vi "lvEtherbone.sdb_find_by_address.vi"(0 "eb_socket_ID":i32, 1 "eb_device_ID":i32, 2 "address":u64 format="%.0x", 5 "error in (no error)":errorcluster) -> (10 "addr_first":u64 format="%.0x", 12 "addr_last":u64 format="%.0x", 13 "eb_status":T1 items=["EB_SUCCESS"=1, "EB_OK"=0, "EB_FAIL"=-1, "EB_ADDRESS"=-2, "EB_WIDTH"=-3, "EB_OVERFLOW"=-4, "EB_ENDIAN"=-5, "EB_BUSY"=-6, "EB_TIMEOUT"=-7, "EB_OOM"=-8, "EB_ABI"=-9, "EB_SEGFAULT"=-10], 14 "eb_socket_ID out":i32, 15 "eb_device_ID out":i32, 16 "vendor_id":u64 format="%.0x", 17 "device_id":u32 format="%.0x", 18 "name":string, 19 "error out":errorcluster)   [LabVIEW 2012, in "lvEtherbone.lvlib"]
doc: "/* Find the SDB record for a device at address.\n * If no matching record is found EB_ADDRESS is returned.\n * On success, EB_OK is returned.\n * Other failures are possible.\n */\nEB_PUBLIC eb_status_t eb_sdb_find_by_address(eb_device_t device, eb_address_t address, struct sdb_device* output);"
uses:
  lvEtherbone.lvlib
  lvEtherbone.lveb_status_t.ctl
  libetherbone.so
panel:
  in  "eb_status_t":T1 items=["EB_SUCCESS"=1, "EB_OK"=0, "EB_FAIL"=-1, "EB_ADDRESS"=-2, "EB_WIDTH"=-3, "EB_OVERFLOW"=-4, "EB_ENDIAN"=-5, "EB_BUSY"=-6, "EB_TIMEOUT"=-7, "EB_OOM"=-8, "EB_ABI"=-9, "EB_SEGFAULT"=-10]
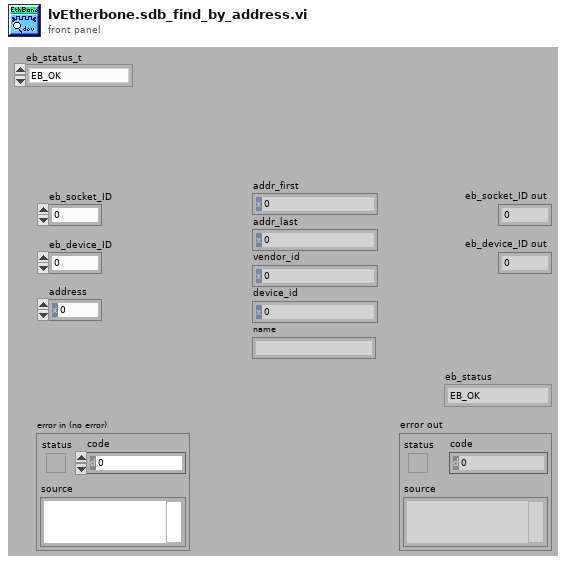
[diagram p1: front panel]
types:
  T1 = typedef "lvEtherbone.lvlib/lvEtherbone.lveb_status_t.ctl" = i32
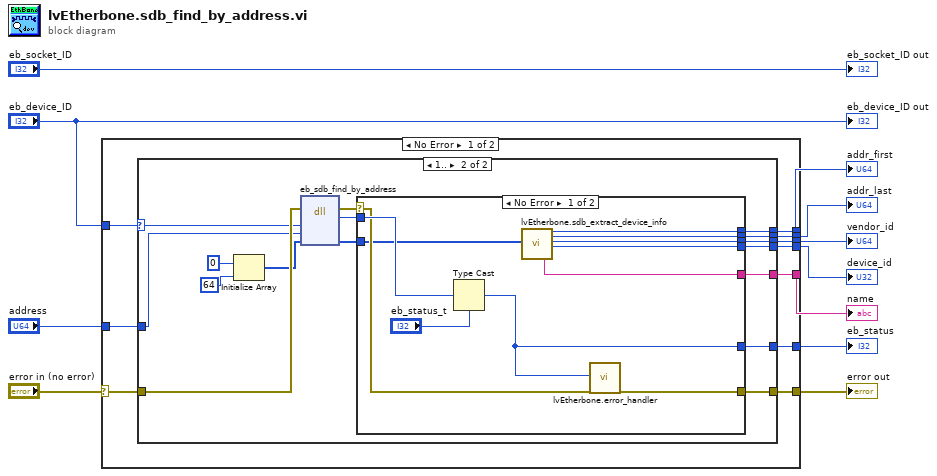
[diagram p0: block diagram]
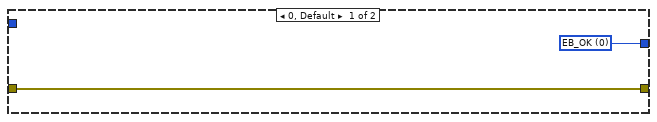
[diagram p2: hidden frame]
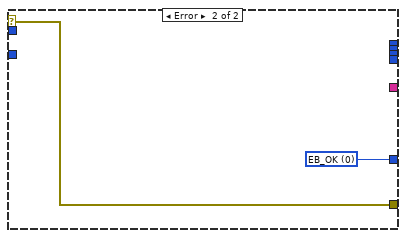
[diagram p3: hidden frame]
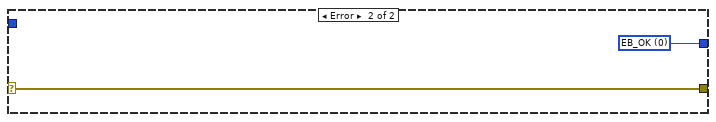
[diagram p4: hidden frame]
diagram:
  n1 = case shown="No Error" "error in (no error)" {
    selector: "error in (no error)" -> [w21 w54]
    tunnel: [w20 w54] -> w10
    tunnel: "address" -> [w18 _]
    tunnel: "eb_device_ID" -> [w17 _]
    tunnel: [w19 w53] -> w8
    tunnel: [w16 _] -> w5
    tunnel: [w15 _] -> w4
    tunnel: [w14 _] -> w3
    tunnel: [w13 _] -> w2
    tunnel: [w12 _] -> w1
    frame No Error {
      n2 = case shown="1.." w17 {
        selector: w17 -> [_ w32]
        tunnel: w21 -> [w22 w37]
        tunnel: [w22 w36] -> w20
        tunnel: [w23 w35] -> w19
        tunnel: w18 -> [_ w33]
        tunnel: [_ w28] -> w16
        tunnel: [_ w27] -> w15
        tunnel: [_ w26] -> w14
        tunnel: [_ w25] -> w13
        tunnel: [_ w24] -> w12
        frame 0, Default {
          w23 = T1 0 items=["EB_SUCCESS"=1, "EB_OK"=0, "EB_FAIL"=-1, "EB_ADDRESS"=-2, "EB_WIDTH"=-3, "EB_OVERFLOW"=-4, "EB_ENDIAN"=-5, "EB_BUSY"=-6, "EB_TIMEOUT"=-7, "EB_OOM"=-8, "EB_ABI"=-9, "EB_SEGFAULT"=-10] ("eb_status_t")
        }
        frame 1.. {
          n3 = Initialize Array(u8 0, 64 ("dimension size")) -> (w29:u8[])
          n4 = dll-call lib="libetherbone.so" fn="eb_sdb_find_by_address"(error in=w37, "device"=w32, "address"=w33, "output"=w29) -> (error out=w38:errorcluster, "eb_status"=w39:i32, "output"=w34:u8[])  [unwired: 4 in, 1 out]
          n5 = case shown="No Error" w38 {
            selector: w38 -> [w47 w52]
            tunnel: w39 -> [w50 _]
            tunnel: [w48 w51] -> w35
            tunnel: [w46 w52] -> w36
            tunnel: w34 -> [w45 _]
            tunnel: [w44 _] -> w28
            tunnel: [w43 _] -> w27
            tunnel: [w42 _] -> w26
            tunnel: [w41 _] -> w25
            tunnel: [w40 _] -> w24
            frame No Error {
              n6 = Type Cast(type="eb_status_t", x=w50) -> (*(type *) &x=w48:T1)
              n7 = call "lvEtherbone.sdb_extract_device_info.vi"("sdb_device_bin"=w45) -> ("name"=w40:string, "addr_first"=w44:u64, "addr_last"=w43:u64, "vendor_id"=w42:u64, "device_id"=w41:u32)  [unwired: 11 in, 3 out]
              n8 = call "lvEtherbone.error_handler.vi"("eb_status"=w48, "error in"=w47) -> ("error out"=w46:errorcluster)  [unwired: 17 in]
            }
            frame Error {
              w51 = T1 0 items=["EB_SUCCESS"=1, "EB_OK"=0, "EB_FAIL"=-1, "EB_ADDRESS"=-2, "EB_WIDTH"=-3, "EB_OVERFLOW"=-4, "EB_ENDIAN"=-5, "EB_BUSY"=-6, "EB_TIMEOUT"=-7, "EB_OOM"=-8, "EB_ABI"=-9, "EB_SEGFAULT"=-10] ("eb_status_t")
            }
          }
        }
      }
    }
    frame Error {
      w53 = T1 0 items=["EB_SUCCESS"=1, "EB_OK"=0, "EB_FAIL"=-1, "EB_ADDRESS"=-2, "EB_WIDTH"=-3, "EB_OVERFLOW"=-4, "EB_ENDIAN"=-5, "EB_BUSY"=-6, "EB_TIMEOUT"=-7, "EB_OOM"=-8, "EB_ABI"=-9, "EB_SEGFAULT"=-10] ("eb_status_t")
    }
  }
  "error out" <- w10
  "eb_status" <- w8
  "addr_first" <- w5
  "addr_last" <- w4
  "device_id" <- w2
  "vendor_id" <- w3
  "name" <- w1
  "eb_socket_ID out" <- "eb_socket_ID"
  "eb_device_ID out" <- "eb_device_ID"
